vi "2D Results to X and Y Arrays.vi"(11 "Results":dbl[][](array[numeric])) -> (2 "Y":dbl[](array[numeric]), 3 "X":dbl[](array[numeric]))   [LabVIEW 2019, in "SMO.Transport.lvclass"]
uses:
  SMO.Transport.lvclass
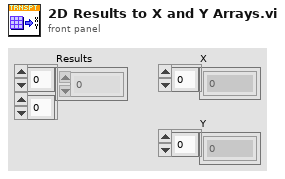
[diagram p1: front panel]
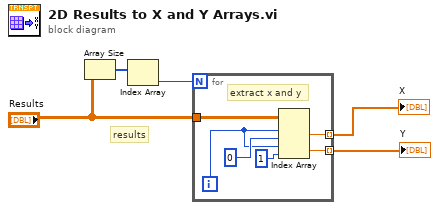
[diagram p0: block diagram]
diagram:
  # "results"
  n1 = Array Size(array="Results") -> (size(s)=w1:i32[])
  n2 = Index Array(array=w1) -> (element=w2:i32)  [unwired: 1 in]
  n3 = for {
    N: w2 -> [_]
    tunnel: "Results" -> [w9]
    tunnel: [w8] -> w4 mode=indexing
    tunnel: [w7] -> w3 mode=indexing
    i -> [w6]
    # "extract x and y"
    n4 = Index Array(array=w9, index (row) #1=w6, index (col) #1=0 ("disabled index (col)"), index (row) #2=w6, index (col) #2=1 ("disabled index (col)")) -> (element #1=w8:dbl, element #2=w7:dbl)
  }
  "X" <- w4
  "Y" <- w3
